vi "Writeprotocol.vi"(8 "error in (no error)":errorcluster, 10 "protocol":string, 11 "object in":refnum<class "kernel_info_reply Message.lvclass">) -> (0 "error out":errorcluster, 3 "object out":refnum<class "kernel_info_reply Message.lvclass">)   [LabVIEW 2018, in "ClientMessaging.lvlib" / "kernel_info_reply Message.lvclass"]
uses:
  kernel_info_reply Message.lvclass
  kernel_info_reply Message.lvclass/kernel_info_reply Message.ctl
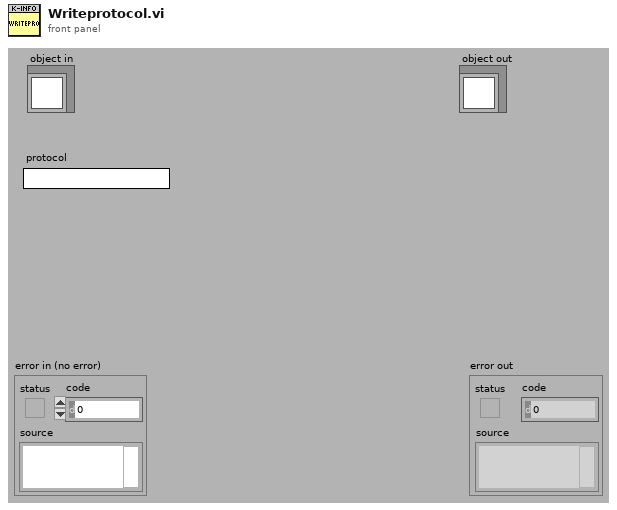
[diagram p1: front panel]
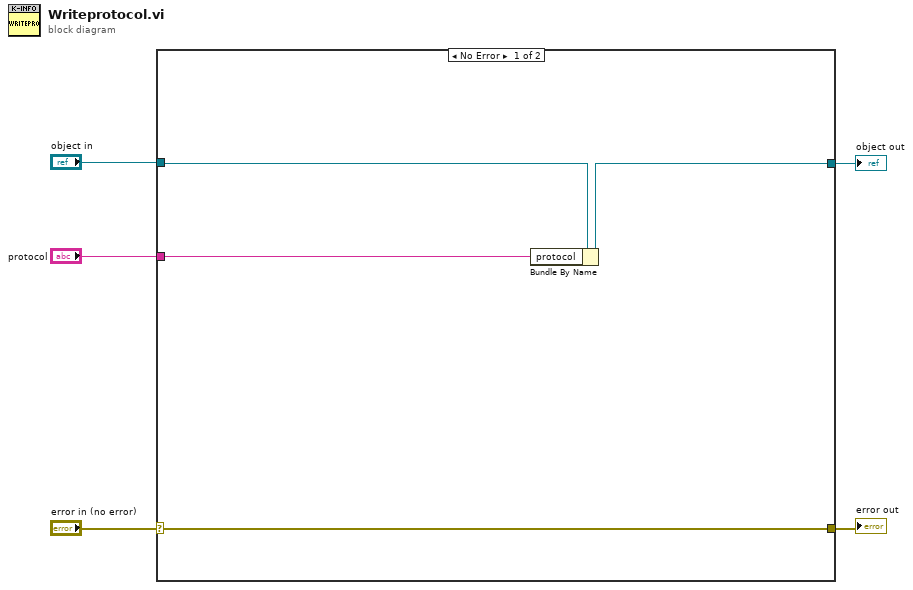
[diagram p0: block diagram]
diagram:
  n1 = case shown="No Error" "error in (no error)" {
    selector: "error in (no error)" -> [w8 w11]
    tunnel: [w8 w11] -> w4
    tunnel: [w6 w10] -> w2
    tunnel: "object in" -> [w7 w10]
    tunnel: "protocol" -> [w9 _]
    frame No Error {
      n2 = Bundle By Name(cluster=w7, "protocol"=w9) -> (w6:refnum<class "kernel_info_reply Message.lvclass">)
    }
    frame Error {
    }
  }
  "error out" <- w4
  "object out" <- w2
